vi "RampToZero.vi"(8 "error in (no error)":errorcluster, 11 "Instrument.VRM in":refnum<class "Instrument.OxfordVRM.lvclass">) -> (0 "error out":errorcluster, 2 "Response":string, 3 "Instrument.VRM out":refnum<class "Instrument.OxfordVRM.lvclass">)   [LabVIEW 2019, in "Instrument.OxfordVRM.lvclass"]
uses:
  Instrument.OxfordVRM.lvclass
  Typedefs/Instrument.VRM.protectedCommands-enum.ctl
  96131257-07af-48a9-a4e4-d10ac3e2b47b.vi
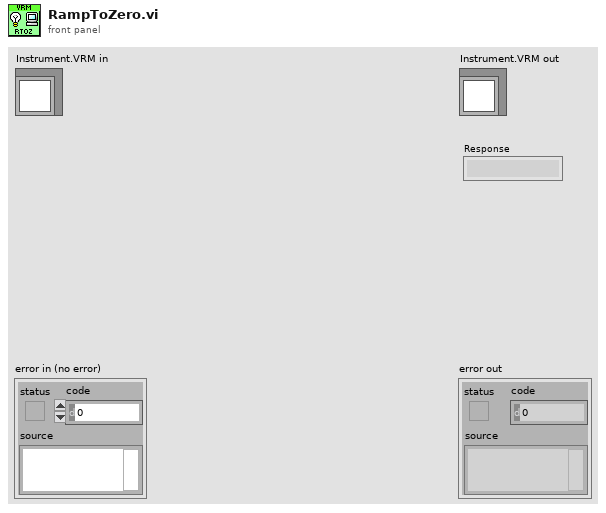
[diagram p1: front panel]
types:
  T1 = typedef "Instrument.OxfordVRM.lvclass/Instrument.VRM.protectedCommands-enum.ctl" = enum16{"Hold", "RampToSet", "RampToZero", "Clamp", "SetTarget", "GetStatus", "GetTarget", "GetField"}
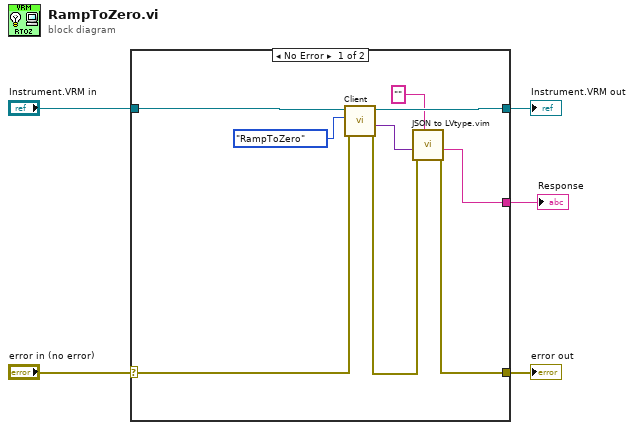
[diagram p0: block diagram]
diagram:
  n1 = case shown="No Error" "error in (no error)" {
    selector: "error in (no error)" -> [w13 w16]
    tunnel: [w11 w16] -> w4
    tunnel: [w12 w15] -> w2
    tunnel: "Instrument.VRM in" -> [w14 w15]
    tunnel: [w10 _] -> w1
    frame No Error {
      n2 = call-dynamic "Client.vi"("error in (no error)"=w13, "Command in"=Instrument.VRM.protectedCommands-enum."RampToZero" ("protectedCommands"), "Instrument in"=w14) -> ("error out"=w6:errorcluster, "Data out"=w8:variant, "Instrument out"=w12:refnum<class "Instrument.OxfordVRM.lvclass">)  [unwired: 5 in, 1 out]
      n3 = call "JSON to LVtype.vim"("type"="", "error in (no error)"=w6, "JSON Data in"=w8) -> ("error out"=w11:errorcluster, "Data out"=w10:string)  [unwired: 7 in]
    }
    frame Error {
    }
  }
  "error out" <- w4
  "Instrument.VRM out" <- w2
  "Response" <- w1
